vi "UI-电源头正面标签露线检测.vi"(8 "error in (no error)":errorcluster caption="错误输入（无错误）", 11 "名称或相对路径":string="Template Program") -> (0 "error in (no error) 2":errorcluster caption="错误输入（无错误）")   [LabVIEW 2017]
uses:
  Picture/SaveButtom.ctl
  Global System.vi
  <vilib>/Utility/xml.llb/Write to XML File(string).vi
panel:
  in  "获取图像":bool
  in  "ROI获取":bool
  in  "创建模板":bool
  in  "保存图像":bool
  out "添加的路径":path
  in  "刷新":bool
  in  "测试按钮":bool
  in  "保存按钮":bool
  in  "Main":enum32{"主参数", "颜色模板匹配参数 ", "测试效果"}(tab)
  in  "UI电源线正面漏线基础参数":T1={"IsNorImage"=TRUE, "Exposure Values"=100289, "ImagePath"=path "C:/Users/hedongpo/Desktop/514-hdp/Alignment Assemble System/Test Picture/B/3.bmp"} caption="参数界面" {"Exposure Values" scale=0.0..200000.0}
  in  "UI电源线正面漏线参数":T3={"Rectangle"={"Left"=0, "Top"=0, "Right"=0, "Bottom"=0, "Rotation"=0.0}, "模板路径"=path "C:/Users/delluser001/Desktop/PowerLine Inspect System/Source Code/Template Program/potteryTemplete/Color.png", "Match Mode "=0, "Minimum Match Score "=800.0, "Number of Matches Requested"=1, "Rotation Angle Ranges (degrees)"=[{"Min"=-180.0, "Max"=180.0}], "Color Sensitivity "=0, "Match Offset"={"X"=0.0, "Y"=0.0}, "Color Score Weight "=500.0, "Search Strategy "=0, "Subpixel Accuracy "=FALSE} {"Rectangle"."Rotation" format="%.2f"; "Rectangle"."Left" scale=0.0..1024.0; "Rectangle"."Right" scale=0.0..1024.0; "Search Strategy" items=["Conservative", "Balance", "Aggressive", "Very Aggressive"]; "Color Sensitivity" items=["Low Sensitivity", "Medium Sensitivity", "High Sensitivity"]; "Match Mode" items=["Shift Invariant", "Rotation Invariant"]}
  out "颜色模板":bool[](array[boolean])
  out "原始图像":T4(plugin-control)
  out "路径输出":path
  in  "Vision Paramter Save Buttom":T5
  out "system time":string
  in  "取消按钮":bool
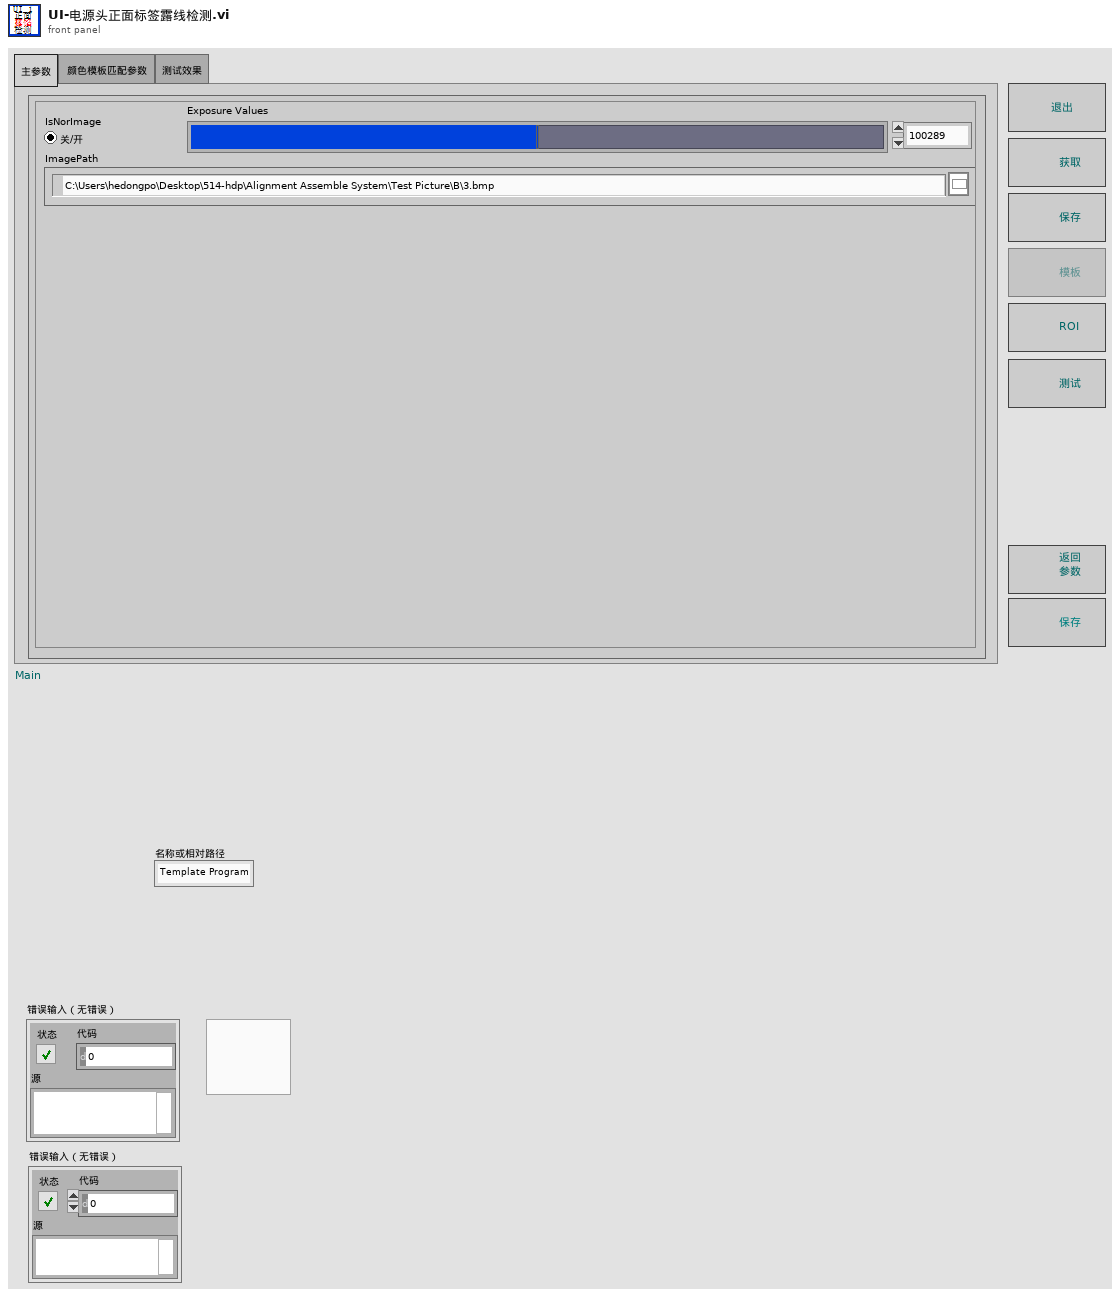
[diagram p1: front panel]
types:
  T1 = cluster{"IsNorImage":bool, "Exposure Values":u32, "ImagePath":path}
  T2 = typedef "IMAQ Rectangle" = cluster{"Left":i32, "Top":i32, "Right":i32, "Bottom":i32, "Rotation":dbl}
  T3 = cluster{"Rectangle":T2, "模板路径":path, "Match Mode ":u32, "Minimum Match Score ":sgl, "Number of Matches Requested":i32, "Rotation Angle Ranges (degrees)":cluster{"Min":sgl, "Max":sgl}[], "Color Sensitivity ":u32, "Match Offset":cluster{"X":sgl, "Y":sgl}, "Color Score Weight ":sgl, "Search Strategy ":u32, "Subpixel Accuracy ":bool}
  T4 = typedef "IMAQ Image.ctl" = refnum<image>
  T5 = typedef "SaveButtom.ctl" = bool
  T6 = cluster{"index":i32, "this vi":refnum<vi>, "error out":errorcluster}
  T7 = cluster{"master data":string, "priority":u16, "secondary data":string[]}
  T8 = cluster{"case name":string[], "queue array":refnum<queue>[]}
  T9 = cluster{"Global Rectangle":i32[], "Contours":cluster{"Contour Type":u32, "ROI Type":u32, "Points":i32[]}[]}
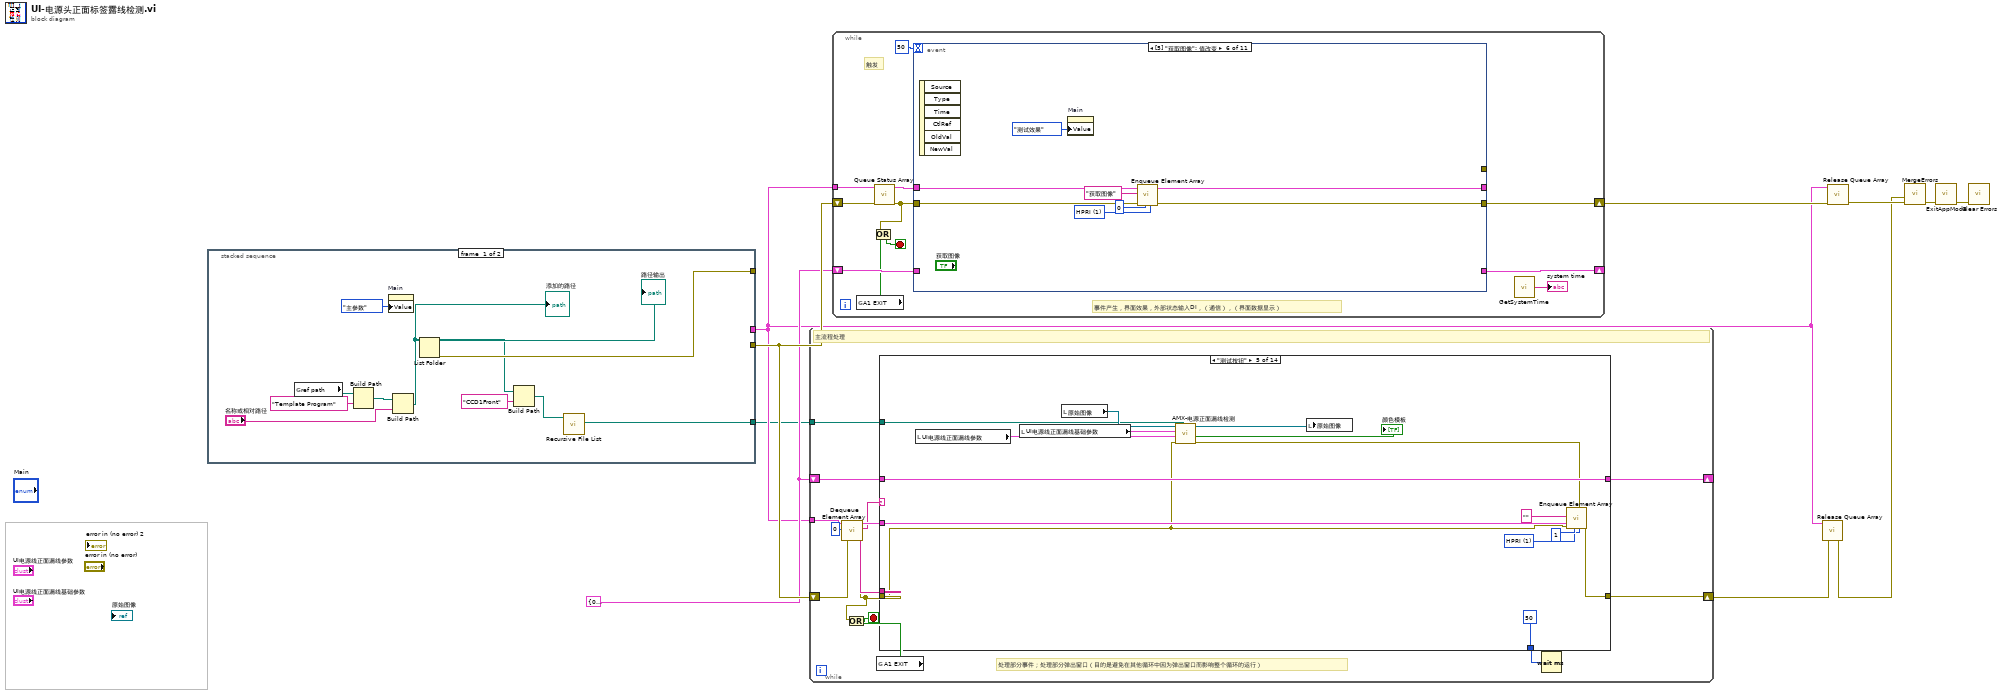
[diagram p0: block diagram]
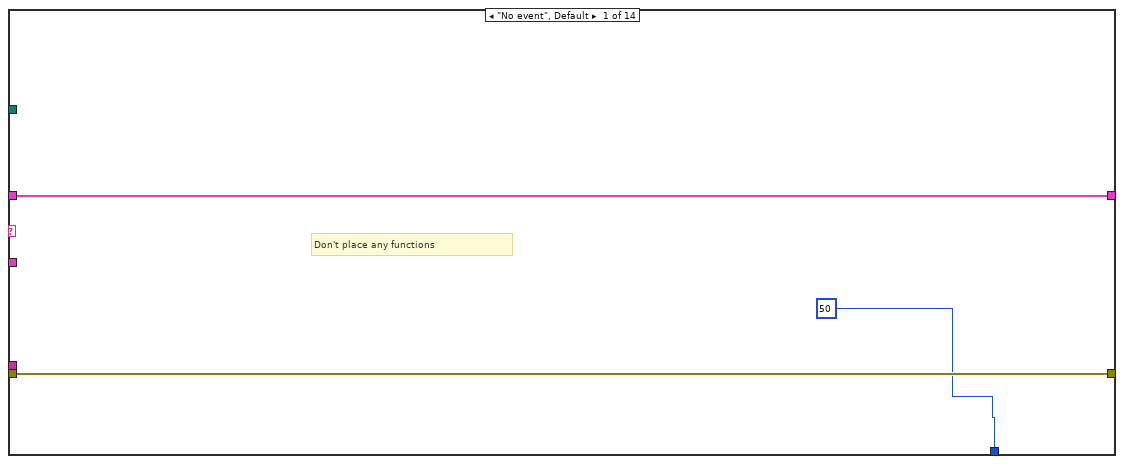
[diagram p2: hidden frame]
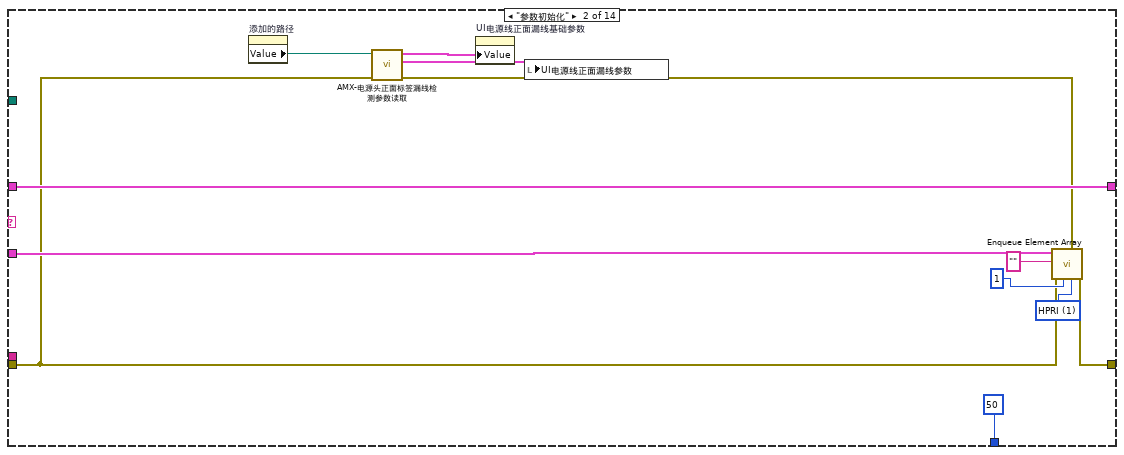
[diagram p3: hidden frame]
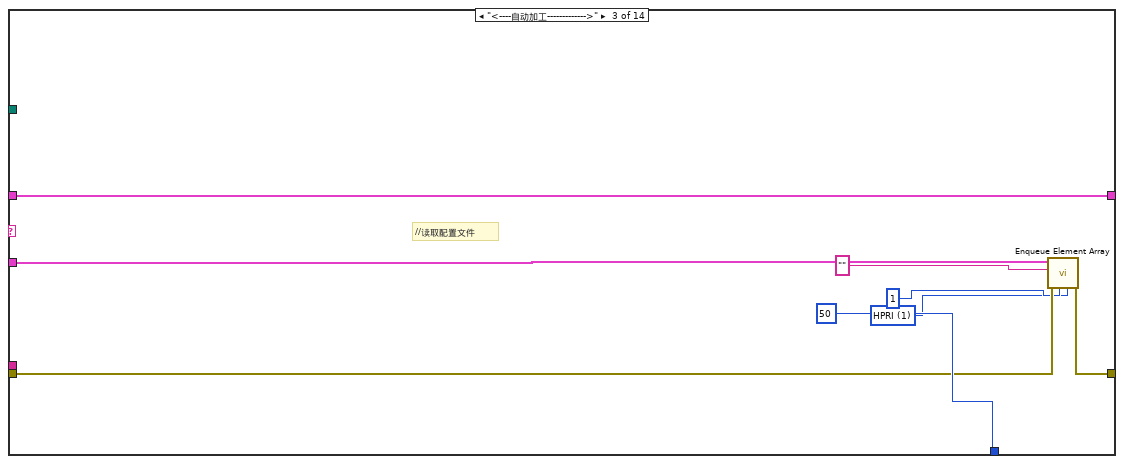
[diagram p4: hidden frame]
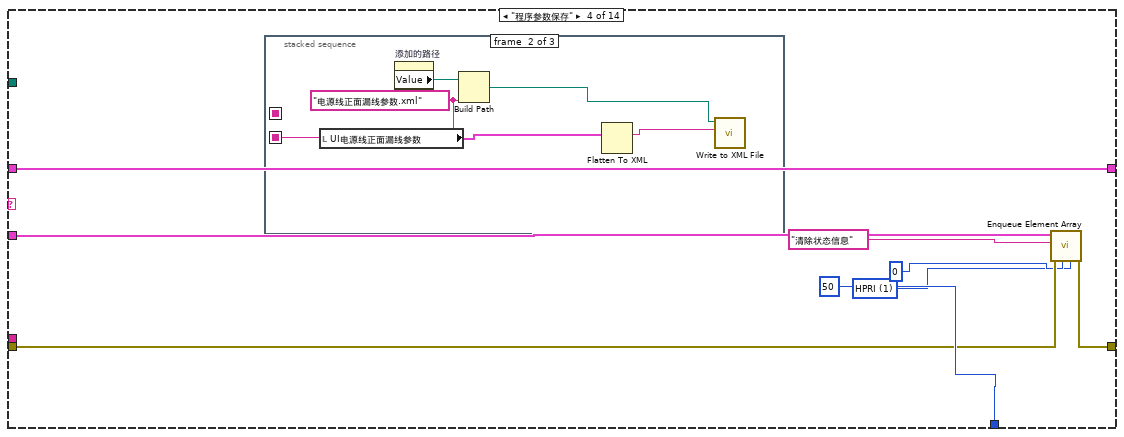
[diagram p5: hidden frame]
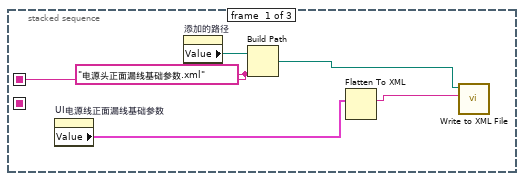
[diagram p6: hidden frame]
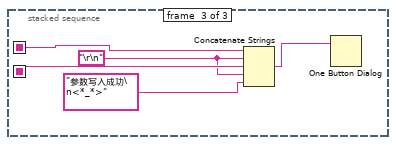
[diagram p7: hidden frame]
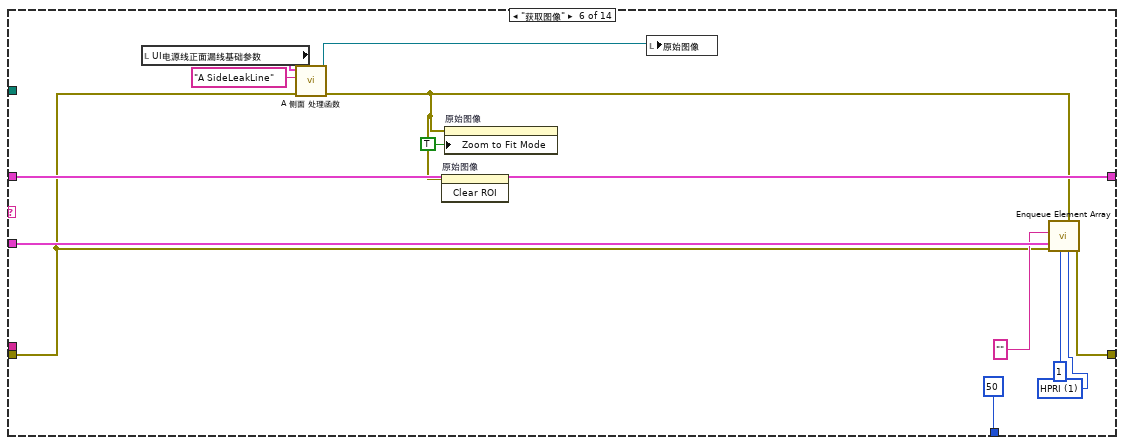
[diagram p8: hidden frame]
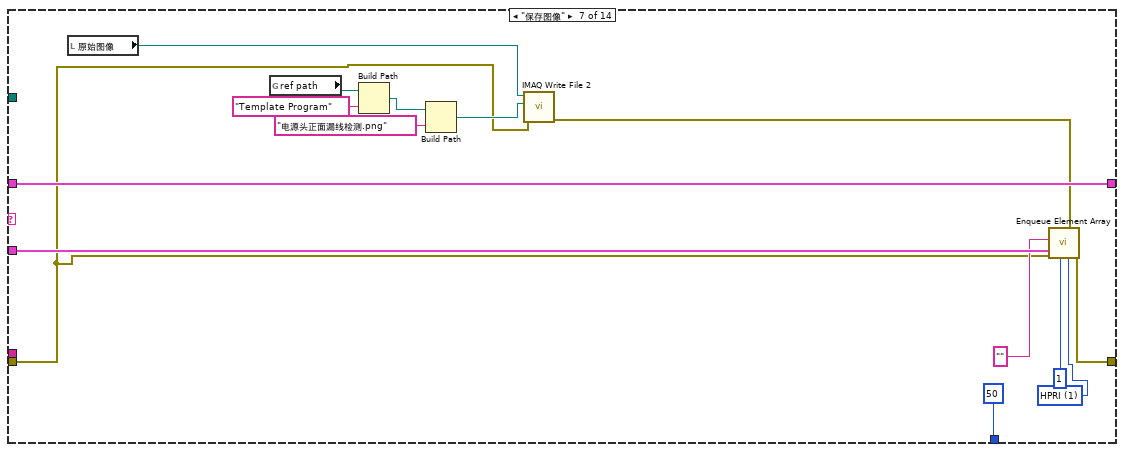
[diagram p9: hidden frame]
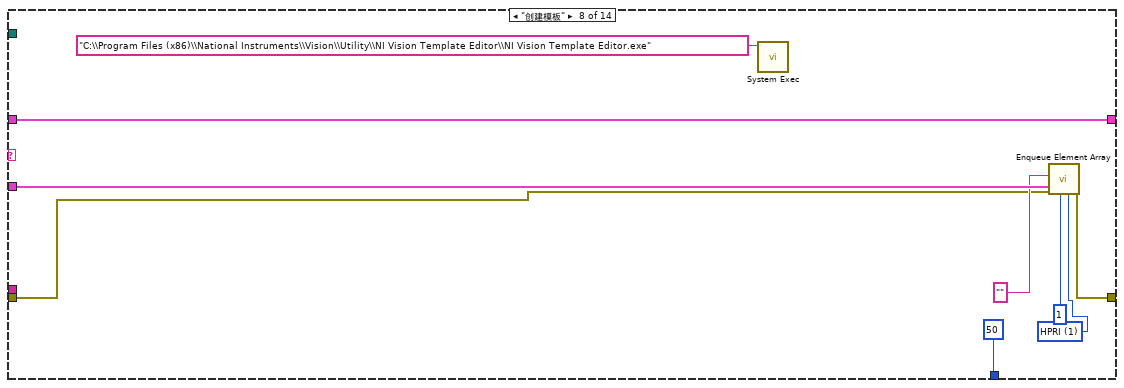
[diagram p10: hidden frame]
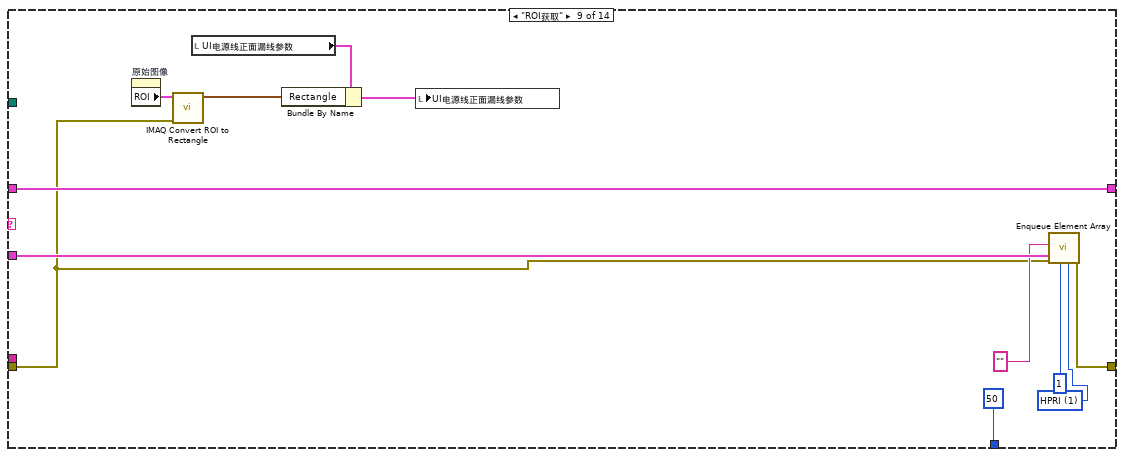
[diagram p11: hidden frame]
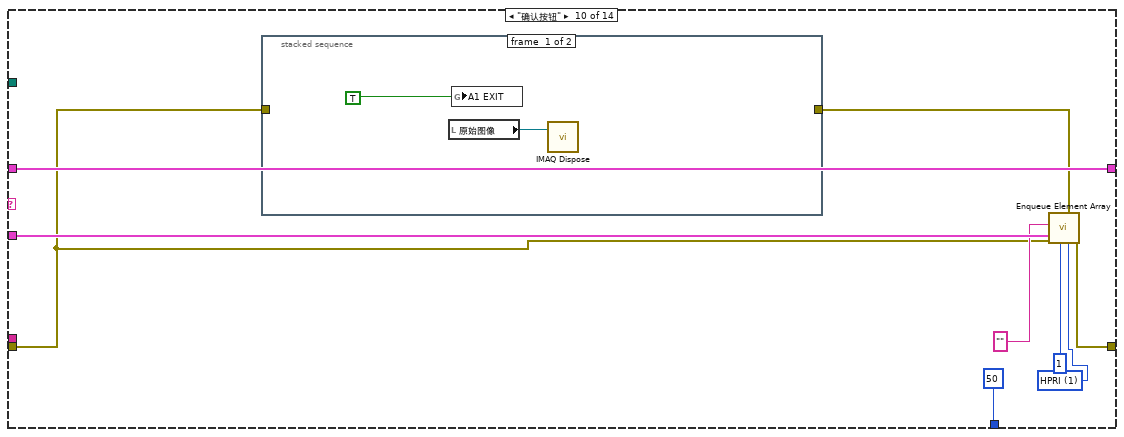
[diagram p12: hidden frame]
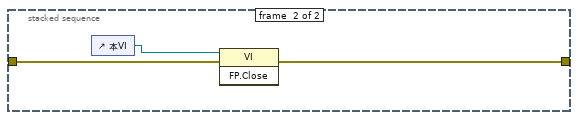
[diagram p13: hidden frame]
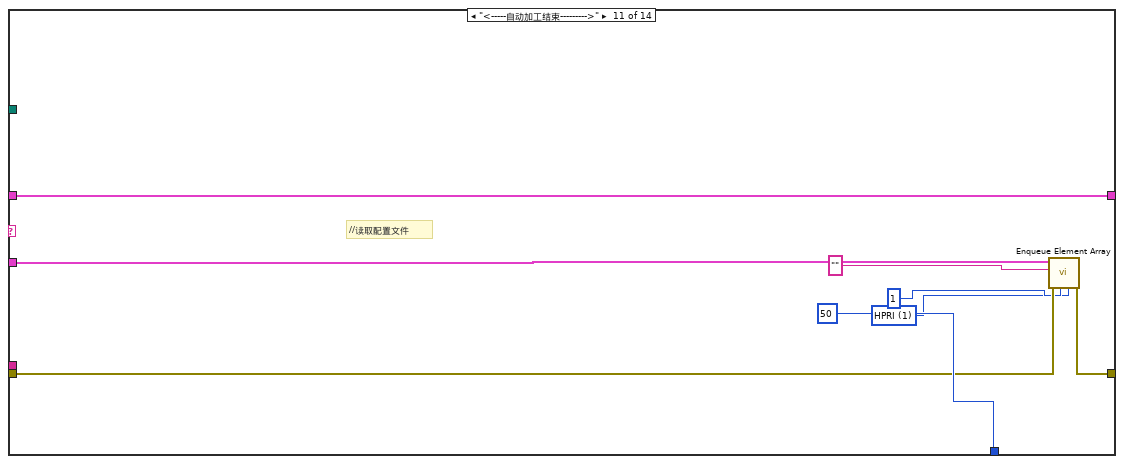
[diagram p14: hidden frame]
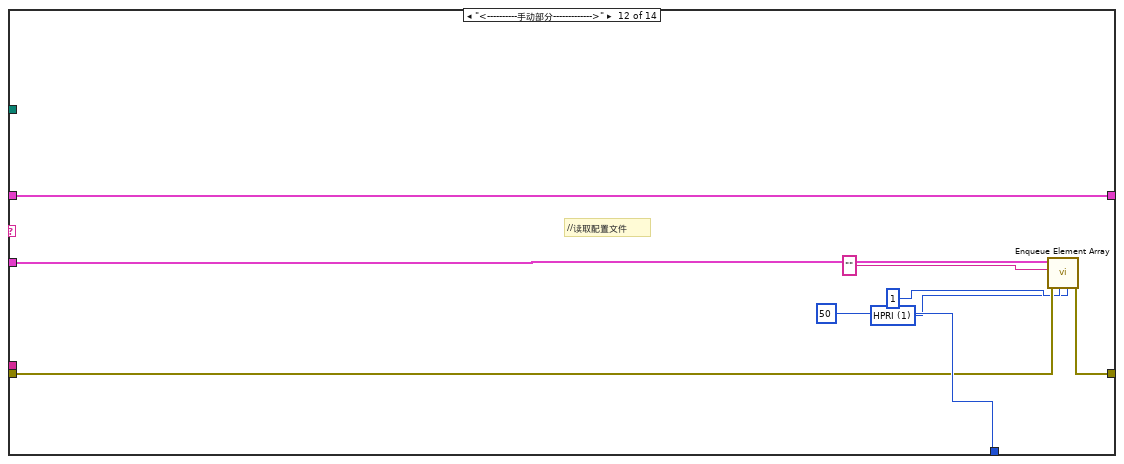
[diagram p15: hidden frame]
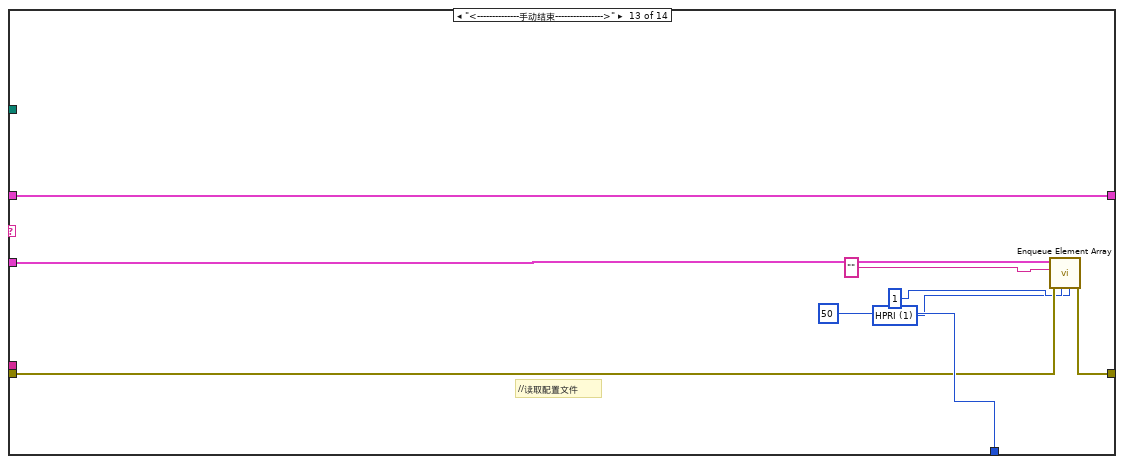
[diagram p16: hidden frame]
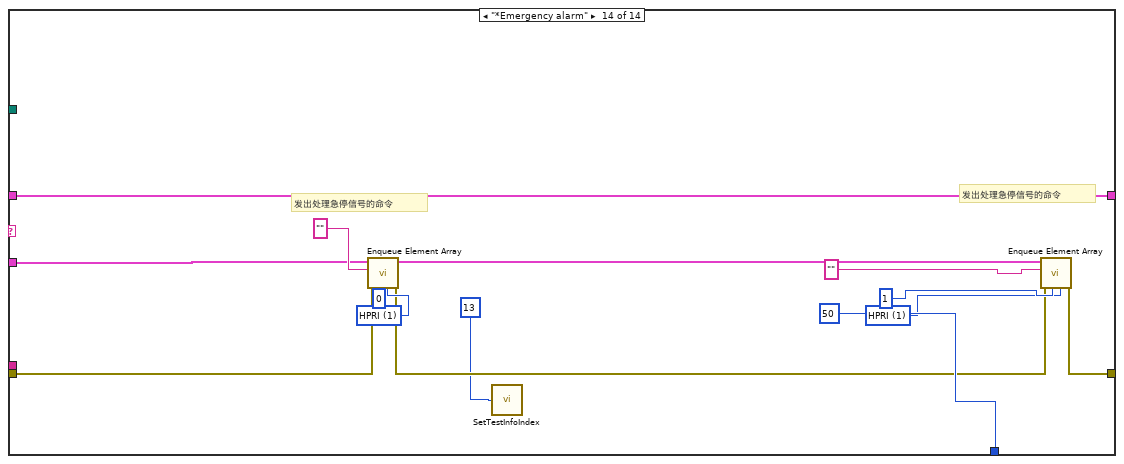
[diagram p17: hidden frame]
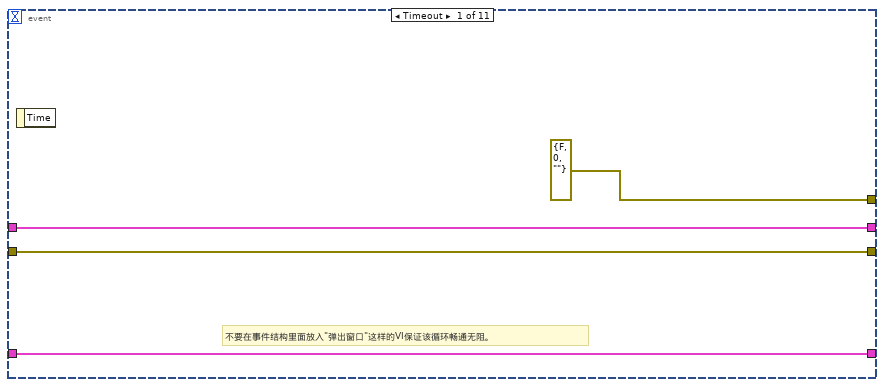
[diagram p18: hidden frame]
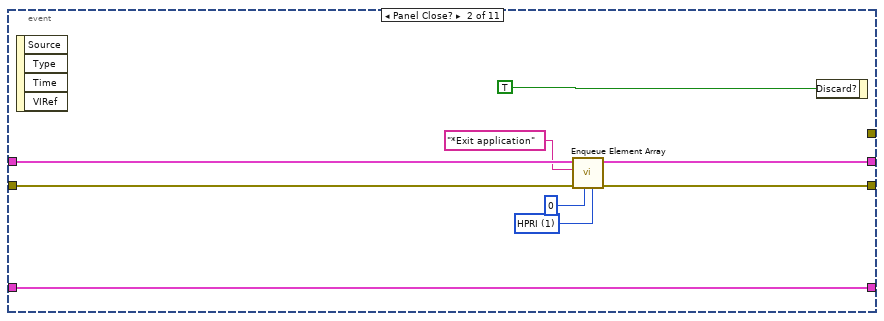
[diagram p19: hidden frame]
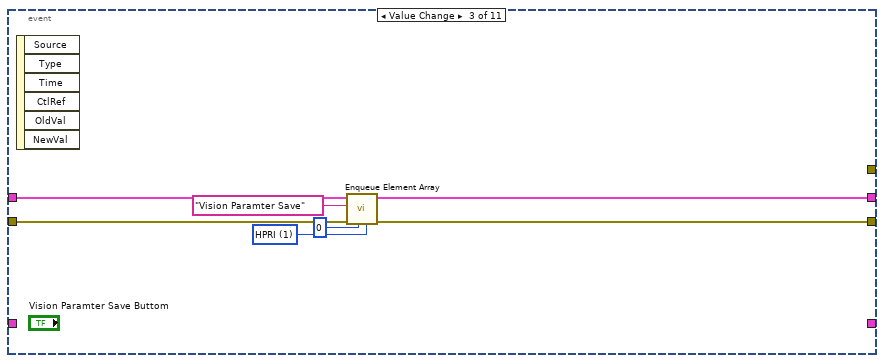
[diagram p20: hidden frame]
diagram:
  w5 = T6 {"index"=0, "this vi"=refnum, "error out"={"status"=FALSE, "code"=0, "source"=""}} ("parameter buffer")
  n1 = stacked-sequence {
    tunnel: [w20 _] -> _
    tunnel: [_ w23] -> w6
    tunnel: [_ w22] -> w2
    tunnel: [w11 _] -> w1
    frame #0 {
      n2 = global read "Global System.vi" "ref path"() -> (w18:path)
      n3 = Build Path(base path=w18, name or relative path="Template Program" ("名称或相对路径")) -> (appended path=w16:path)
      n4 = property on="Main" class="TabCtl (严格)"("Value"=enum32{"主参数", "颜色模板匹配参数 ", "测试效果"}."主参数" ("Main")) -> ()  [unwired: 2 in, 2 out]
      n5 = Build Path(base path=w16, name or relative path="名称或相对路径") -> (appended path=w12:path)
      "添加的路径" <- w12
      n6 = List Folder(path=w12) -> (path out=→"路径输出":path, error out=w20:errorcluster)  [unwired: 3 in, 2 out]
      n7 = Build Path(base path=w12, name or relative path="CCD1Front" ("名称或相对路径")) -> (appended path=w13:path)
      n8 = call <vilib>:"Recursive File List.vi"("Folder Path"=w13) -> ("All Files in Dir"=w11:path[])  [unwired: 6 in, 4 out]
    }
    frame #1 {
      w31 = string[] ["comm queue1", "data queue 11", "data queue 12", "data queue 13", "data queue 14"]  # queue name
      w32 = 4  # queue num
      w33 = T7 {"master data"="", "priority"=0, "secondary data"=[]}  # element data type
      n9 = call "Obtain Queue Array.vi"("queue name"=w31, "element data type"=w33, "queue num"=w32) -> ("error out"=w27:errorcluster, "queue out"=w28:T8)  [unwired: 2 in, 1 out]
      n10 = call "Enqueue Element Array.vi"("queue index"=0, "error in"=w27, "master data"="参数初始化", "queue in"=w28) -> ("error out"=w26:errorcluster, "queue out"=w25:T8)  [unwired: 6 in]
      n11 = disable-structure shown="启用" {
        disable-tunnel: w26 -> [w39 w40]
        disable-tunnel: w25 -> [w38 w41]
        disable-tunnel: "Loading Variable" ("master data") -> [w37 _]
        disable-tunnel: [w35 w40] -> w23
        disable-tunnel: [w34 w41] -> w22
        frame Disabled {
          n12 = call "Enqueue Element Array.vi"("queue index"=12, "error in"=w39, "master data"=w37, "queue in"=w38) -> ("error out"=w35:errorcluster, "queue out"=w34:T8)  [unwired: 6 in]
        }
        frame Enabled {
        }
      }
    }
  }
  n13 = while {
    shift-right: [w55] -> w4
    shift-left: w6 -> [w46]
    shift-right: [w52] -> _
    shift-left: w5 -> [w53]
    tunnel: w2 -> [w48]
    tunnel: w1 -> [w42]
    stop <- w43 stop-if-true
    # "处理部分事件；处理部分弹出窗口（目的是避免在其他循环中因为弹出窗口而影响整个循环的运行）"
    # "主流程处理"
    n14 = call "Dequeue Element Array.vi"("queue in"=w48, "queue index"=0, "error in"=w46) -> ("queue out"=w51:T8, "master data"=w50:string, "secondary data"=w49:string[], "error out"=w45:errorcluster)  [unwired: 2 in, 1 out]
    n15 = global read "Global System.vi" "A1 EXIT"() -> (w44:bool)
    n16 = Or(x=w45, y=w44) -> (x .or. y?=w43:bool)
    n17 = case shown="\"测试按钮\"" w50 {
      tunnel: w51 -> [_ w69 w77 w79 w115 w128 w143 w152 w164 w173 w186 w194 w202 w208]
      tunnel: w45 -> [w57 w62 w73 w83 w108 w119 w130 w146 w157 w167 w182 w190 w198 w205]
      tunnel: [w57 w68 w76 w85 w114 w127 w142 w151 w163 w172 w185 w193 w201 w216] -> w55
      tunnel: [50 50 50 50 50 50 50 50 50 50 50 50 50 50] -> w54
      tunnel: w53 -> [w58 w64 w74 w80 w110 w123 w138 w147 w159 w168 w183 w191 w199 w214]
      tunnel: [w58 w64 w74 w80 w110 w123 w138 w147 w159 w168 w183 w191 w199 w214] -> w52
      tunnel: w49 -> [_ _ _ _ _ _ _ _ _ _ _ _ _ _]
      tunnel: w42 -> [_ _ _ _ w103 _ _ _ _ _ _ _ _ _]
      frame "No event", Default {
        # "Don't place any functions"
      }
      frame "参数初始化" {
        w65 = u16 1 items=["HPRI"=1, "LPRI"=0] ("priority")
        n18 = property on="添加的路径" class="Path"() -> ("Value"=w63:path)  [unwired: 2 in, 2 out]
        n19 = call "AMX-电源头正面标签漏线检测参数读取.vi"("error in (no error)"=w62, "基路径"=w63) -> ("error out"=w60:errorcluster, "UI电源线正面漏线参数"=w59:T3, "UI电源线正面漏线基础参数"=w61:T1)  [unwired: 6 in]
        n20 = property on="UI电源线正面漏线基础参数" class="Clust (严格)"("Value"=w61) -> ()  [unwired: 2 in, 2 out]
        n21 = local write "UI电源线正面漏线参数"(w59) -> ()
        n22 = call "Enqueue Element Array.vi"("priority"=w65, "device error in"=w60, "queue index"=1, "error in"=w62, "master data"="" ("Element 1"), "queue in"=w69) -> ("error out"=w68:errorcluster)  [unwired: 4 in, 1 out]
      }
      frame "<----自动加工------------->" {
        w71 = u16 1 items=["HPRI"=1, "LPRI"=0] ("priority")
        # "//读取配置文件"
        n23 = call "Enqueue Element Array.vi"("priority"=w71, "queue index"=1, "error in"=w73, "master data"="" ("Element 1"), "queue in"=w77) -> ("error out"=w76:errorcluster)  [unwired: 5 in, 1 out]
      }
      frame "程序参数保存" {
        w81 = u16 1 items=["HPRI"=1, "LPRI"=0] ("priority")
        n24 = stacked-sequence {
          seq-local: [w87 _ _] -> [_ _ w100]
          seq-local: [_ w93 _] -> [_ _ w98]
          frame #0 {
            w87 = "电源头正面漏线基础参数.xml" ("名称或相对路径")
            n25 = property on="UI电源线正面漏线基础参数" class="Clust (严格)"() -> ("Value"=w90:T1)  [unwired: 2 in, 2 out]
            n26 = property on="添加的路径" class="Path"() -> ("Value"=w91:path)  [unwired: 2 in, 2 out]
            n27 = Build Path(base path=w91, name or relative path=w87) -> (appended path=w88:path)
            n28 = Flatten To XML(anything=w90) -> (xml string=w89:string)
            n29 = call-poly <vilib>:"Write to XML File.vi"("XML Input"=w89, "XML File Path"=w88) -> ()  [unwired: 7 in, 3 out]
          }
          frame #1 {
            w93 = "电源线正面漏线参数.xml" ("名称或相对路径")
            n30 = local read "UI电源线正面漏线参数"() -> (w92:T3)
            n31 = property on="添加的路径" class="Path"() -> ("Value"=w96:path)  [unwired: 2 in, 2 out]
            n32 = Build Path(base path=w96, name or relative path=w93) -> (appended path=w94:path)
            n33 = Flatten To XML(anything=w92) -> (xml string=w95:string)
            n34 = call-poly <vilib>:"Write to XML File.vi"("XML Input"=w95, "XML File Path"=w94) -> ()  [unwired: 7 in, 3 out]
          }
          frame #2 {
            w97 = "\r\n"
            n35 = Concatenate Strings(w100, w97, w98, w97, "参数写入成功\n<*_*>" ("消息")) -> (w99:string)
            n36 = One Button Dialog(message=w99) -> ()  [unwired: 1 in, 1 out]
          }
        }
        n37 = call "Enqueue Element Array.vi"("priority"=w81, "queue index"=0, "error in"=w83, "master data"="清除状态信息" ("Element 1"), "queue in"=w79) -> ("error out"=w85:errorcluster)  [unwired: 5 in, 1 out]
      }
      frame "测试按钮" {
        w111 = u16 1 items=["HPRI"=1, "LPRI"=0] ("priority")
        n38 = local read "UI电源线正面漏线参数"() -> (w104:T3)
        n39 = local read "UI电源线正面漏线基础参数"() -> (w109:T1)
        n40 = local read "原始图像"() -> (w106:T4)
        n41 = call "AMX-电源正面漏线检测.vi"("模板路径"=w103, "error in (no error)"=w108, "UI电源线正面漏线参数"=w104, "电源线正面标签1基础参数"=w109, "Image in"=w106) -> ("error out"=w105:errorcluster, "结果"=→"颜色模板":bool[], "Image out"=w107:T4)  [unwired: 1 in, 3 out]
        n42 = local write "原始图像"(w107) -> ()
        n43 = call "Enqueue Element Array.vi"("priority"=w111, "device error in"=w105, "queue index"=1, "error in"=w108, "master data"="" ("Element 1"), "queue in"=w115) -> ("error out"=w114:errorcluster)  [unwired: 4 in, 1 out]
      }
      frame "获取图像" {
        w124 = u16 1 items=["HPRI"=1, "LPRI"=0] ("priority")
        n44 = local read "UI电源线正面漏线基础参数"() -> (w121:T1)
        n45 = call "A 侧面 处理函数.vi"("error in (no error)"=w119, "Image Name"="A SideLeakLine", "ParamsUI"=w121) -> ("error out"=w117:errorcluster, "Image out"=w120:T4)  [unwired: 5 in, 2 out]
        n46 = invoke on="原始图像" class="ImageControl" method="Clear ROI"(error in=w117) -> ()  [unwired: 2 in, 3 out]
        n47 = property on="原始图像" class="ImageControl"(error in=w117, "Zoom to Fit Mode"=TRUE) -> ()  [unwired: 1 in, 2 out]
        n48 = local write "原始图像"(w120) -> ()
        n49 = call "Enqueue Element Array.vi"("priority"=w124, "device error in"=w117, "queue index"=1, "error in"=w119, "master data"="" ("Element 1"), "queue in"=w128) -> ("error out"=w127:errorcluster)  [unwired: 4 in, 1 out]
      }
      frame "保存图像" {
        w139 = u16 1 items=["HPRI"=1, "LPRI"=0] ("priority")
        n50 = local read "原始图像"() -> (w131:T4)
        n51 = global read "Global System.vi" "ref path"() -> (w137:path)
        n52 = Build Path(base path=w137, name or relative path="Template Program" ("名称或相对路径")) -> (appended path=w135:path)
        n53 = Build Path(base path=w135, name or relative path="电源头正面漏线检测.png" ("名称或相对路径")) -> (appended path=w133:path)
        n54 = call-poly "IMAQ Write File 2"("error in (no error)"=w130, "File Path"=w133, "Image"=w131) -> ("error out"=w132:errorcluster)  [unwired: 7 in, 1 out]
        n55 = call "Enqueue Element Array.vi"("priority"=w139, "device error in"=w132, "queue index"=1, "error in"=w130, "master data"="" ("Element 1"), "queue in"=w143) -> ("error out"=w142:errorcluster)  [unwired: 4 in, 1 out]
      }
      frame "创建模板" {
        w148 = u16 1 items=["HPRI"=1, "LPRI"=0] ("priority")
        n56 = call <vilib>:"System Exec.vi"("command line"="C:\\Program Files (x86)\\National Instruments\\Vision\\Utility\\NI Vision Template Editor\\NI Vision Template Editor.exe") -> ()  [unwired: 7 in, 4 out]
        n57 = call "Enqueue Element Array.vi"("priority"=w148, "queue index"=1, "error in"=w146, "master data"="" ("Element 1"), "queue in"=w152) -> ("error out"=w151:errorcluster)  [unwired: 5 in, 1 out]
      }
      frame "ROI获取" {
        w160 = u16 1 items=["HPRI"=1, "LPRI"=0] ("priority")
        n58 = property on="原始图像" class="ImageControl"() -> ("ROI"=w158:T9)  [unwired: 2 in, 2 out]
        n59 = call "IMAQ Convert ROI to Rectangle"("error in (no error)"=w157, "ROI Descriptor"=w158) -> ("Rectangle"=w155:T2)  [unwired: 7 in, 1 out]
        n60 = local read "UI电源线正面漏线参数"() -> (w156:T3)
        n61 = Bundle By Name(cluster=w156, "Rectangle"=w155) -> (w154:T3)
        n62 = local write "UI电源线正面漏线参数"(w154) -> ()
        n63 = call "Enqueue Element Array.vi"("priority"=w160, "queue index"=1, "error in"=w157, "master data"="" ("Element 1"), "queue in"=w164) -> ("error out"=w163:errorcluster)  [unwired: 5 in, 1 out]
      }
      frame "确认按钮" {
        w169 = u16 1 items=["HPRI"=1, "LPRI"=0] ("priority")
        n64 = stacked-sequence {
          tunnel: w167 -> [_ w178]
          tunnel: [_ w177] -> w166
          frame #0 {
            n65 = local read "原始图像"() -> (w175:T4)
            n66 = global write "Global System.vi" "A1 EXIT"(TRUE ("EXIT")) -> ()
            n67 = call "IMAQ Dispose"("Image"=w175) -> ()  [unwired: 5 in, 1 out]
          }
          frame #1 {
            n68 = control-ref of="本VI"() -> (w179:refnum<vi>)
            n69 = invoke class="VI" method="FP.Close"(reference=w179, error in=w178) -> (error out=w177:errorcluster)  [unwired: 1 in, 2 out]
          }
        }
        n70 = call "Enqueue Element Array.vi"("priority"=w169, "device error in"=w166, "queue index"=1, "error in"=w167, "master data"="" ("Element 1"), "queue in"=w173) -> ("error out"=w172:errorcluster)  [unwired: 4 in, 1 out]
      }
      frame "<-----自动加工结束--------->" {
        w180 = u16 1 items=["HPRI"=1, "LPRI"=0] ("priority")
        # "//读取配置文件"
        n71 = call "Enqueue Element Array.vi"("priority"=w180, "queue index"=1, "error in"=w182, "master data"="" ("Element 1"), "queue in"=w186) -> ("error out"=w185:errorcluster)  [unwired: 5 in, 1 out]
      }
      frame "<----------手动部分------------->" {
        w188 = u16 1 items=["HPRI"=1, "LPRI"=0] ("priority")
        # "//读取配置文件"
        n72 = call "Enqueue Element Array.vi"("priority"=w188, "queue index"=1, "error in"=w190, "master data"="" ("Element 1"), "queue in"=w194) -> ("error out"=w193:errorcluster)  [unwired: 5 in, 1 out]
      }
      frame "<--------------手动结束---------------->" {
        w196 = u16 1 items=["HPRI"=1, "LPRI"=0] ("priority")
        # "//读取配置文件"
        n73 = call "Enqueue Element Array.vi"("priority"=w196, "queue index"=1, "error in"=w198, "master data"="" ("Element 1"), "queue in"=w202) -> ("error out"=w201:errorcluster)  [unwired: 5 in, 1 out]
      }
      frame "*Emergency alarm" {
        w211 = u16 1 items=["HPRI"=1, "LPRI"=0] ("priority")
        w212 = u16 1 items=["HPRI"=1, "LPRI"=0] ("priority")
        # "发出处理急停信号的命令"
        # "发出处理急停信号的命令"
        n74 = call "Enqueue Element Array.vi"("priority"=w211, "queue index"=0, "error in"=w205, "master data"="" ("Element 1"), "queue in"=w208) -> ("error out"=w206:errorcluster, "queue out"=w207:T8)  [unwired: 5 in]
        n75 = call "SetTestInfoIndex.vi"("test info index"=13) -> ()
        n76 = call "Enqueue Element Array.vi"("priority"=w212, "queue index"=1, "error in"=w206, "master data"="" ("Element 1"), "queue in"=w207) -> ("error out"=w216:errorcluster)  [unwired: 5 in, 1 out]
      }
    }
    n77 = Wait (ms)(milliseconds to wait=w54) -> ()  [unwired: 1 out]
  }
  n78 = while {
    shift-right: [w221] -> w7
    shift-left: w6 -> [w225]
    shift-right: [w223] -> _
    shift-left: w5 -> [w224]
    tunnel: w2 -> [w227]
    stop <- w218 stop-if-true
    # "触发"
    # "事件产生，界面效果，外部状态输入DI，（通信），（界面数据显示）"
    n79 = global read "Global System.vi" "A1 EXIT"() -> (w219:bool)
    n80 = call "Queue Status Array.vi"("error in (no error)"=w225, "queue in"=w227) -> ("error out"=w220:errorcluster, "queue out"=w222:T8)  [unwired: 4 in]
    n81 = Or(x=w220, y=w219) -> (x .or. y?=w218:bool)
    n82 = event shown="[5] \"获取图像\": 值改变" {
      selector: _ -> [_ _ _ _ _ _ _ _ _ _ _]
      dyn-events: _ -> [_ _ _ _ _ _ _ _ _ _ _]
      timeout: 50 -> [_ _ _ _ _ _ _ _ _ _ _]
      tunnel: w224 -> [w232 w240 _ _ _ _ _ _ _ _ _]
      tunnel: [w232 w240 _ _ _ _ _ _ _ _ _] -> w223
      tunnel: [errorcluster {"status"=FALSE, "code"=0, "source"=""} ("error out") _ _ _ _ _ _ _ _ _ _] -> _
      tunnel: w222 -> [w230 w239 w245 w252 w259 w267 w274 w281 w289 w297 w305]
      tunnel: w220 -> [w229 w238 w244 w251 w258 w266 w273 w280 w288 w296 w304]
      tunnel: [w229 w237 w242 w249 w256 w264 w271 w278 w286 w294 w302] -> w221
      tunnel: [w230 w236 w243 w250 w257 w265 w272 w279 w287 w295 w303] -> _
      event Timeout {
        # "不要在事件结构里面放入\"弹出窗口\"这样的VI保证该循环畅通无阻。"
        n83 = event-data() -> ()  [unwired: 1 in, 1 out]
      }
      event Panel Close? {
        w234 = u16 1 items=["HPRI"=1, "LPRI"=0] ("priority")
        n84 = event-data() -> ()  [unwired: 1 in, 4 out]
        n85 = call "Enqueue Element Array.vi"("priority"=w234, "queue index"=0, "error in"=w238, "master data"="*Exit application", "queue in"=w239) -> ("error out"=w237:errorcluster, "queue out"=w236:T8)  [unwired: 5 in]
        n86 = event-data("Discard?"=TRUE) -> ()  [unwired: 1 in, 1 out]
      }
      event Value Change {
        w247 = u16 1 items=["HPRI"=1, "LPRI"=0] ("priority")
        n87 = event-data() -> ()  [unwired: 1 in, 6 out]
        n88 = call "Enqueue Element Array.vi"("priority"=w247, "queue index"=0, "error in"=w244, "master data"="Vision Paramter Save", "queue in"=w245) -> ("error out"=w242:errorcluster, "queue out"=w243:T8)  [unwired: 5 in]
      }
      event "取消按钮": Value Change {
        w254 = u16 1 items=["HPRI"=1, "LPRI"=0] ("priority")
        n89 = event-data() -> ()  [unwired: 1 in, 6 out]
        n90 = call "Enqueue Element Array.vi"("priority"=w254, "queue index"=0, "error in"=w251, "master data"="确认按钮", "queue in"=w252) -> ("error out"=w249:errorcluster, "queue out"=w250:T8)  [unwired: 5 in]
      }
      event "保存按钮": Value Change {
        w261 = u16 1 items=["HPRI"=1, "LPRI"=0] ("priority")
        n91 = event-data() -> ()  [unwired: 1 in, 6 out]
        n92 = call "Enqueue Element Array.vi"("priority"=w261, "queue index"=0, "error in"=w258, "master data"="程序参数保存", "queue in"=w259) -> ("error out"=w256:errorcluster, "queue out"=w257:T8)  [unwired: 5 in]
      }
      event "获取图像": Value Change {
        w269 = u16 1 items=["HPRI"=1, "LPRI"=0] ("priority")
        n93 = event-data() -> ()  [unwired: 1 in, 6 out]
        n94 = property on="Main" class="TabCtl (严格)"("Value"=enum32{"主参数", "颜色模板匹配参数 ", "测试效果"}."测试效果" ("Main")) -> ()  [unwired: 2 in, 2 out]
        n95 = call "Enqueue Element Array.vi"("priority"=w269, "queue index"=0, "error in"=w266, "master data"="获取图像", "queue in"=w267) -> ("error out"=w264:errorcluster, "queue out"=w265:T8)  [unwired: 5 in]
      }
      event "保存图像": Value Change {
        w276 = u16 1 items=["HPRI"=1, "LPRI"=0] ("priority")
        n96 = event-data() -> ()  [unwired: 1 in, 6 out]
        n97 = call "Enqueue Element Array.vi"("priority"=w276, "queue index"=0, "error in"=w273, "master data"="保存图像", "queue in"=w274) -> ("error out"=w271:errorcluster, "queue out"=w272:T8)  [unwired: 5 in]
      }
      event "创建模板": Value Change {
        w283 = u16 1 items=["HPRI"=1, "LPRI"=0] ("priority")
        n98 = event-data() -> ()  [unwired: 1 in, 6 out]
        n99 = call "Enqueue Element Array.vi"("priority"=w283, "queue index"=0, "error in"=w280, "master data"="创建模板", "queue in"=w281) -> ("error out"=w278:errorcluster, "queue out"=w279:T8)  [unwired: 5 in]
      }
      event "ROI获取": Value Change {
        w291 = u16 1 items=["HPRI"=1, "LPRI"=0] ("priority")
        n100 = event-data() -> ()  [unwired: 1 in, 6 out]
        n101 = property on="Main" class="TabCtl (严格)"("Value"=enum32{"主参数", "颜色模板匹配参数 ", "测试效果"}."颜色模板匹配参数 " ("Main")) -> ()  [unwired: 2 in, 2 out]
        n102 = call "Enqueue Element Array.vi"("priority"=w291, "queue index"=0, "error in"=w288, "master data"="ROI获取", "queue in"=w289) -> ("error out"=w286:errorcluster, "queue out"=w287:T8)  [unwired: 5 in]
      }
      event "测试按钮": Value Change {
        w299 = u16 1 items=["HPRI"=1, "LPRI"=0] ("priority")
        n103 = event-data() -> ()  [unwired: 1 in, 6 out]
        n104 = property on="Main" class="TabCtl (严格)"("Value"=enum32{"主参数", "颜色模板匹配参数 ", "测试效果"}."测试效果" ("Main")) -> ()  [unwired: 2 in, 2 out]
        n105 = call "Enqueue Element Array.vi"("priority"=w299, "queue index"=0, "error in"=w296, "master data"="测试按钮", "queue in"=w297) -> ("error out"=w294:errorcluster, "queue out"=w295:T8)  [unwired: 5 in]
      }
      event "刷新": Value Change {
        n106 = event-data() -> ()  [unwired: 1 in, 6 out]
        n107 = disable-structure shown="禁用" {
          disable-tunnel: w305 -> [w309 _]
          disable-tunnel: w304 -> [w308 _]
          disable-tunnel: [w307 _] -> w303
          disable-tunnel: [w306 _] -> w302
          frame Disabled {
            w311 = u16 1 items=["HPRI"=1, "LPRI"=0] ("priority")
            # "刷新"
            n108 = call "Enqueue Element Array.vi"("priority"=w311, "queue index"=0, "error in"=w308, "master data"="刷新", "queue in"=w309) -> ("error out"=w306:errorcluster, "queue out"=w307:T8)  [unwired: 5 in]
          }
          frame Enabled {
          }
        }
        n109 = property on="Main" class="TabCtl (严格)"("Value"=enum32{"主参数", "颜色模板匹配参数 ", "测试效果"}."颜色模板匹配参数 " ("Main")) -> ()  [unwired: 2 in, 2 out]
      }
    }
    n110 = call "GetSystemTime.vi"() -> ("date/time string"=→"system time":string)  [unwired: 7 in]
  }
  n111 = call "Release Queue Array.vi"("error in"=w4, "queue in"=w2) -> ("error out"=w3:errorcluster)  [unwired: 2 in, 3 out]
  n112 = call "Release Queue Array.vi"("error in"=w7, "queue in"=w2) -> ("error out"=w10:errorcluster)  [unwired: 2 in, 3 out]
  n113 = call "MergeErrors.vi"("error in 3 (no error)"=w3, "error in 4 (no error)"=w10) -> ("error out"=w9:errorcluster)  [unwired: 6 in]
  n114 = call "ExitAppMode.vi"("error in (no error)"=w9) -> ("error out"=w8:errorcluster)  [unwired: 10 in]
  n115 = call <vilib>:"Clear Errors.vi"("error in (no error)"=w8) -> ()  [unwired: 5 in, 2 out]
